vi "Cool Until Target.vi"(8 "error in (no error)":errorcluster, 10 "target temperature":dbl[unit]=273.15, 11 "cooling system in":refnum<class "Compressor Cooler.lvclass">) -> (0 "error out":errorcluster, 3 "cooling system out":refnum<class "Compressor Cooler.lvclass">)   [LabVIEW 2023, in "Compressor Cooler.lvclass"]
uses:
  Compressor Cooler.lvclass
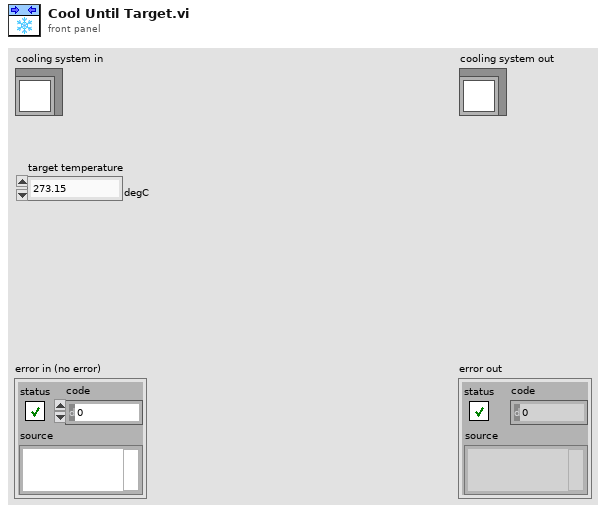
[diagram p1: front panel]
types:
  T1 = enum16{"Suck", "Compress", "Blow", "Decompress"}[]
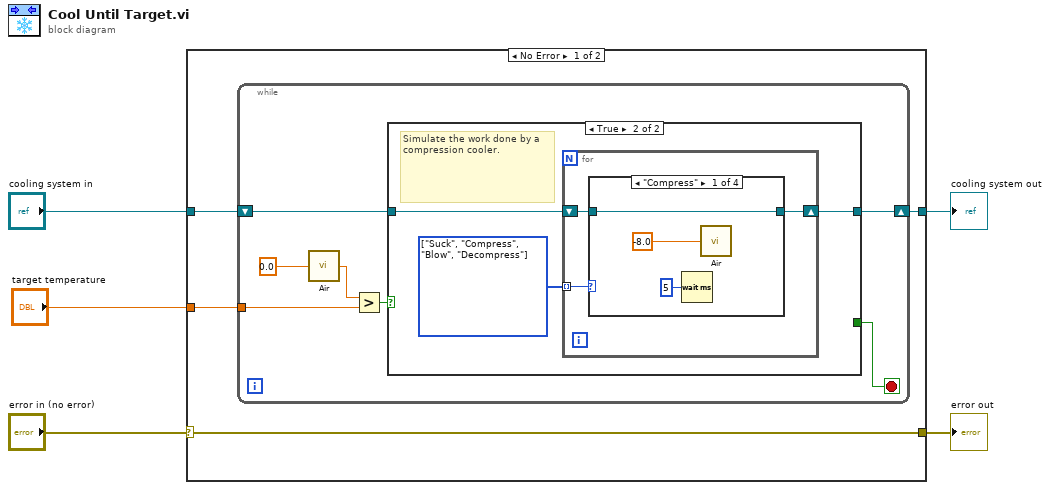
[diagram p0: block diagram]
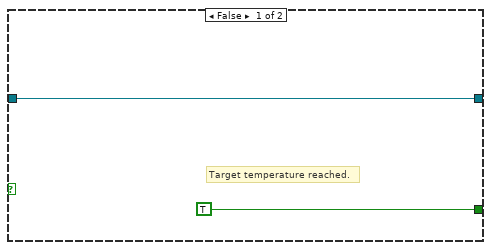
[diagram p2: hidden frame]
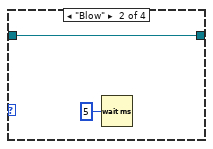
[diagram p3: hidden frame]
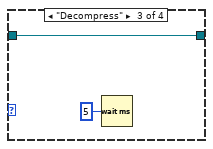
[diagram p4: hidden frame]
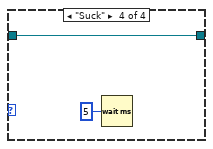
[diagram p5: hidden frame]
diagram:
  n1 = case shown="No Error" "error in (no error)" {
    selector: "error in (no error)" -> [w9 w35]
    tunnel: "target temperature" -> [w8 _]
    tunnel: [w9 w35] -> w3
    tunnel: [w7 w34] -> w2
    tunnel: "cooling system in" -> [w6 w34]
    frame No Error {
      n2 = while {
        tunnel: w8 -> [w14]
        shift-right: [w11] -> w7
        shift-left: w6 -> [w10]
        stop <- w12 stop-if-true
        n3 = call "Air.vi"("temperature adjustment"=dbl[unit] 0.0) -> ("new air temperature"=w15:dbl[unit])
        n4 = Greater?(x=w15, y=w14) -> (0:w13:bool)
        n5 = case shown="True" w13 {
          tunnel: [TRUE _] -> w12
          tunnel: [w17 w20] -> w11
          tunnel: w10 -> [w17 w19]
          frame False {
            # "Target temperature reached."
          }
          frame True {
            w21 = T1 [enum."Suck", enum."Compress", enum."Blow", enum."Decompress"] items=["Suck", "Compress", "Blow", "Decompress"]
            # "Simulate the work done by a compression cooler."
            n6 = for {
              tunnel: w21 -> [w24] mode=indexing
              shift-right: [w23] -> w20
              shift-left: w19 -> [w22]
              n7 = case shown="\"Compress\"" w24 {
                tunnel: [w25 w28 w30 w32] -> w23
                tunnel: w22 -> [w25 w28 w30 w32]
                frame "Compress" {
                  n8 = Wait (ms)(milliseconds to wait=u32 5) -> ()  [unwired: 1 out]
                  n9 = call "Air.vi"("temperature adjustment"=dbl[unit] -8.0) -> ()  [unwired: 1 out]
                }
                frame "Blow" {
                  n10 = Wait (ms)(milliseconds to wait=u32 5) -> ()  [unwired: 1 out]
                }
                frame "Decompress" {
                  n11 = Wait (ms)(milliseconds to wait=u32 5) -> ()  [unwired: 1 out]
                }
                frame "Suck" {
                  n12 = Wait (ms)(milliseconds to wait=u32 5) -> ()  [unwired: 1 out]
                }
              }
            }
          }
        }
      }
    }
    frame Error {
    }
  }
  "error out" <- w3
  "cooling system out" <- w2
